vi "Parse Response.vi"(5 "Headers":string, 7 "Body":string, 11 "error in (no error)":errorcluster) -> (4 "Response Code":i32, 15 "error out":errorcluster)   [LabVIEW 2020, in "VolatusGUIElements.lvlib" / "HttpButtonControl.lvclass"]
uses:
  HttpButtonControl.lvclass
  HttpButtonControl.lvclass/HttpButtonControl.ctl
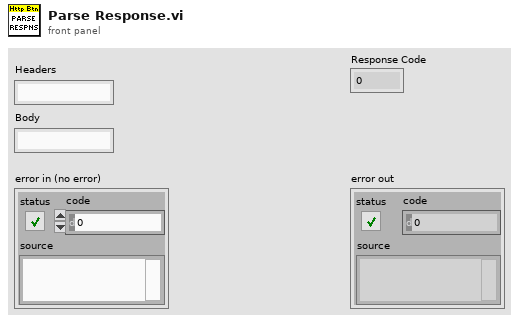
[diagram p1: front panel]
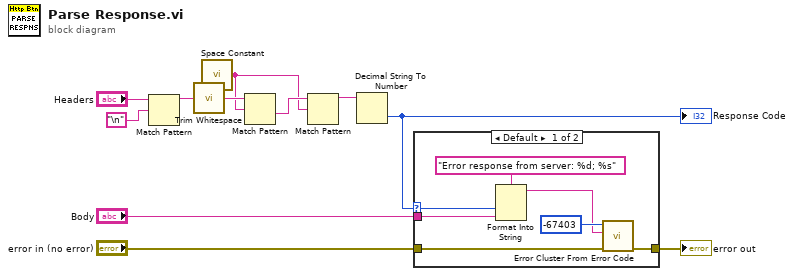
[diagram p0: block diagram]
diagram:
  n1 = Match Pattern(string="Headers", regular expression="\n") -> (before substring=w9:string)  [unwired: 1 in, 3 out]
  n2 = call <vilib>:"Trim Whitespace.vi"("string"=w9) -> ("trimmed string"=w8:string)  [unwired: 1 in]
  n3 = call <vilib>:"Space Constant.vi"() -> ("String"=w6:string)
  n4 = Match Pattern(string=w8, regular expression=w6) -> (after substring=w7:string)  [unwired: 1 in, 3 out]
  n5 = Match Pattern(string=w7, regular expression=w6) -> (before substring=w5:string)  [unwired: 1 in, 3 out]
  n6 = Decimal String To Number(string=w5) -> (number=w4:i32)  [unwired: 2 in, 1 out]
  "Response Code" <- w4
  n7 = case shown="Default" w4 {
    selector: w4 -> [w14 _]
    tunnel: "error in (no error)" -> [w18 w19]
    tunnel: [w17 w19] -> w2
    tunnel: "Body" -> [w13 _]
    frame Default {
      n8 = Format Into String(format string="Error response from server: %d; %s", w14, w13) -> (resulting string=w12:string)  [unwired: 2 in, 1 out]
      n9 = call <vilib>:"Error Cluster From Error Code.vi"("error in (no error)"=w18, "error message (\"\")"=w12, "error code (0)"=-67403) -> ("error out"=w17:errorcluster)  [unwired: 6 in]
    }
    frame 200..299 {
    }
  }
  "error out" <- w2
